vi "Get Default UIPs.vi"() -> (2 "UIPs":refnum<class "UIP.lvclass">[](array[class]))   [LabVIEW 2015, in "UIM.lvclass"]
doc: "Returns a list of all default UIPs used by the UIM. This can be used to more easily point to the inbuilt UIPs when loading new UIPs."
uses:
  UIM.lvclass
  UIP/UIP.lvclass
  Plugin UIPs/TipStripUIP/TipStripUIP.lvclass
  Plugin UIPs/DescriptionUIP/DescriptionUIP.lvclass
  Plugin UIPs/VisibleUIP/VisibleUIP.lvclass
  Plugin UIPs/SizeUIP/SizeUIP.lvclass
  Plugin UIPs/DisabledUIP/DisabledUIP.lvclass
  Plugin UIPs/PositionUIP/PositionUIP.lvclass
  Plugin UIPs/CaptionUIP/CaptionUIP.lvclass
  Plugin UIPs/ValueUIP/ValueUIP.lvclass
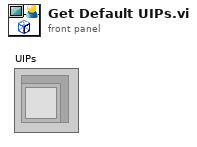
[diagram p1: front panel]
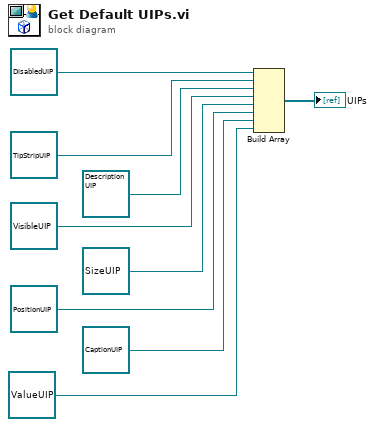
[diagram p0: block diagram]
diagram:
  n1 = Build Array(refnum<class "DisabledUIP.lvclass"> refnum ("DisabledUIP.lvclass"), refnum<class "TipStripUIP.lvclass"> refnum ("TipStripUIP.lvclass"), refnum<class "DescriptionUIP.lvclass"> refnum ("DescriptionUIP.lvclass"), refnum<class "VisibleUIP.lvclass"> refnum ("VisibleUIP.lvclass"), refnum<class "SizeUIP.lvclass"> refnum ("SizeUIP.lvclass"), refnum<class "PositionUIP.lvclass"> refnum ("PositionUIP.lvclass"), refnum<class "CaptionUIP.lvclass"> refnum ("CaptionUIP.lvclass"), refnum<class "ValueUIP.lvclass"> refnum ("ValueUIP.lvclass")) -> (→"UIPs":refnum<class "UIP.lvclass">[])
